vi "Send Message.vi"(8 "error in (no error)":errorcluster, 10 "TestManagerMsg":refnum<class "TestManagerMsg.lvclass">, 11 "Properties in":refnum<class "Properties.lvclass">) -> (0 "error out":errorcluster, 3 "Properties out":refnum<class "Properties.lvclass">)   [LabVIEW 2013, in "Caraya.lvlib" / "Properties.lvclass"]
uses:
  Properties.lvclass
  Test Manager Message/TestManagerMsg.lvclass
  Properties.lvclass/Properties.ctl
  Basic Test Manager/Basic Test Manager.lvclass
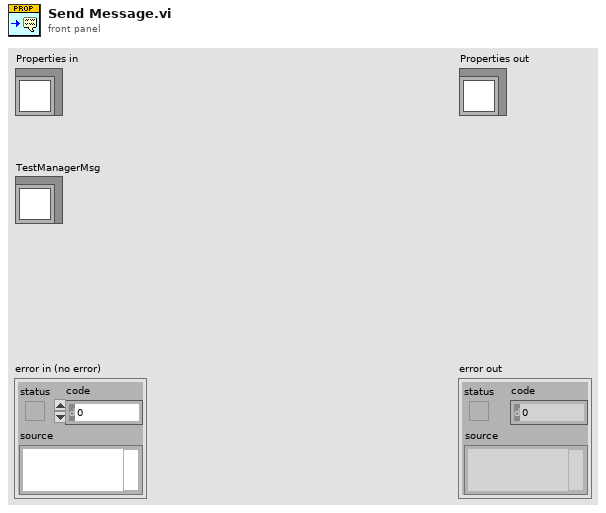
[diagram p1: front panel]
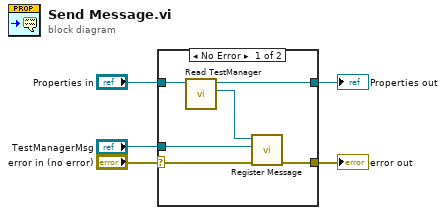
[diagram p0: block diagram]
diagram:
  n1 = case shown="No Error" "error in (no error)" {
    selector: "error in (no error)" -> [w7 w13]
    tunnel: [w6 w13] -> w4
    tunnel: [w9 w12] -> w2
    tunnel: "Properties in" -> [w10 w12]
    tunnel: "TestManagerMsg" -> [w8 _]
    frame No Error {
      n2 = call "Read TestManager.vi"("Properties in"=w10) -> ("Test Manager"=w11:refnum<class "Basic Test Manager.lvclass">, "Properties out"=w9:refnum<class "Properties.lvclass">)  [unwired: 9 in]
      n3 = call-dynamic "Register Message.vi"("error in (no error)"=w7, "TestManagerMsg"=w8, "Basic Test Manager in"=w11) -> ("error out"=w6:errorcluster)  [unwired: 7 in, 1 out]
    }
    frame Error {
    }
  }
  "error out" <- w4
  "Properties out" <- w2
